vi "Create Routine.vi"(8 "error in (no error)":errorcluster, 10 "Routine":T1 {"Stop Parameters"."Response"."Byte Order" items=["Little Endian", "Big Endian"]; "Stop Parameters"."Response"."Data Type" items=["Signed", "Unsigned", "IEEE Float"]; "Stop Parameters"."Cmd"."Byte Order" items=["Little Endian", "Big Endian"]; "Stop Parameters"."Cmd"."Data Type" items=["Signed", "Unsigned", "IEEE Float"]; "Request Parameters"."Response"."Byte Order" items=["Little Endian", "Big Endian"]; "Request Parameters"."Response"."Data Type" items=["Signed", "Unsigned", "IEEE Float"]; "Request Parameters"."Cmd"."Byte Order" items=["Little Endian", "Big Endian"]; "Request Parameters"."Cmd"."Data Type" items=["Signed", "Unsigned", "IEEE Float"]; "Start Parameters"."Response"."Byte Order" items=["Little Endian", "Big Endian"]; "Start Parameters"."Response"."Data Type" items=["Signed", "Unsigned", "IEEE Float"]; "Start Parameters"."Cmd"."Byte Order" items=["Little Endian", "Big Endian"]; "Start Parameters"."Cmd"."Data Type" items=["Signed", "Unsigned", "IEEE Float"]}, 11 "Section Ptr":T4 format="%.0x") -> (0 "error out":errorcluster, 3 "Parent Ref out":T4 format="%.0x")   [LabVIEW 2015, in "Diagnostics Addon System Explorer.lvlib"]
uses:
  System Explorer/Diagnostics Addon System Explorer.lvlib
  <vilib>/NI Veristand/Custom Device API/Custom Device Item Ref.ctl
  Routine Paramaters.ctl
  Input and Output Signal Parameters.ctl
  Signal Parameters.ctl
  FG Action.ctl
  GUID Lookup.vi
  <vilib>/NI Veristand/Custom Device API/NI VeriStand - Get Item Property.vi
  <vilib>/NI Veristand/Custom Device API/Get Item Property (U32).vi
  <vilib>/NI Veristand/Custom Device API/NI VeriStand - Set Item Property.vi
  <vilib>/NI Veristand/Custom Device API/Set Item Property (U32).vi
  <vilib>/NI Veristand/Custom Device API/Custom Device API.lvlib
  Diagnostics Addon Shared.lvlib
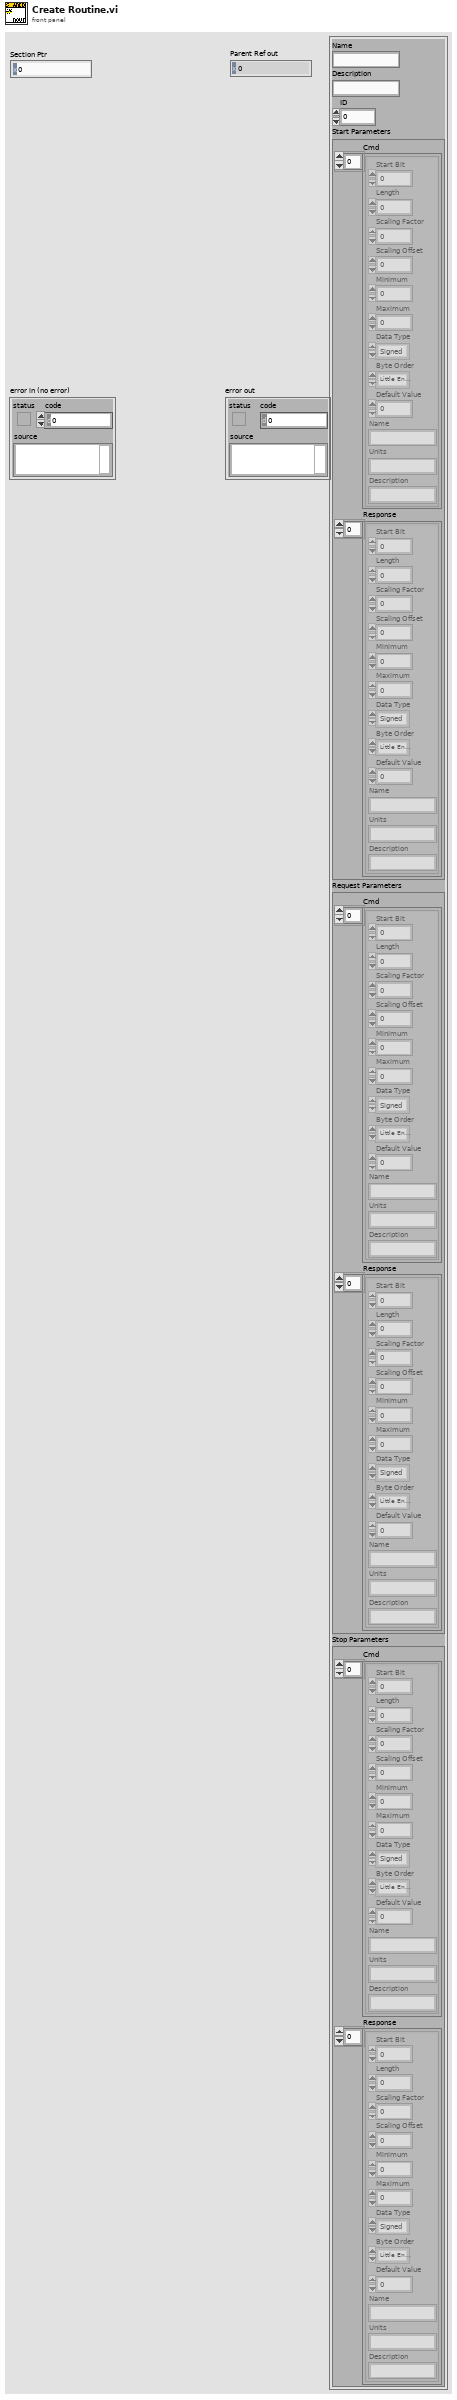
[diagram p1: front panel]
types:
  T1 = typedef "Diagnostics Addon Shared.lvlib/Routine Paramaters.ctl" = cluster{"Name":string, "Description":string, "ID":u16, "Start Parameters":T2, "Request Parameters":T2, "Stop Parameters":T2}
  T2 = typedef "Diagnostics Addon Shared.lvlib/Input and Output Signal Parameters.ctl" = cluster{"Cmd":T3[], "Response":T3[]}
  T3 = typedef "Diagnostics Addon Shared.lvlib/Signal Parameters.ctl" = cluster{"Start Bit":u8, "Length":u8, "Scaling Factor":dbl, "Scaling Offset":dbl, "Minimum":dbl, "Maximum":dbl, "Data Type":u32, "Byte Order":u32, "Default Value":dbl, "Name":string, "Units":string, "Description":string}
  T4 = typedef "Custom Device API.lvlib/Custom Device Item Ref.ctl" = u64
  T5 = typedef "Diagnostics Addon System Explorer.lvlib/FG Action.ctl" = enum16{"Get", "Set"}
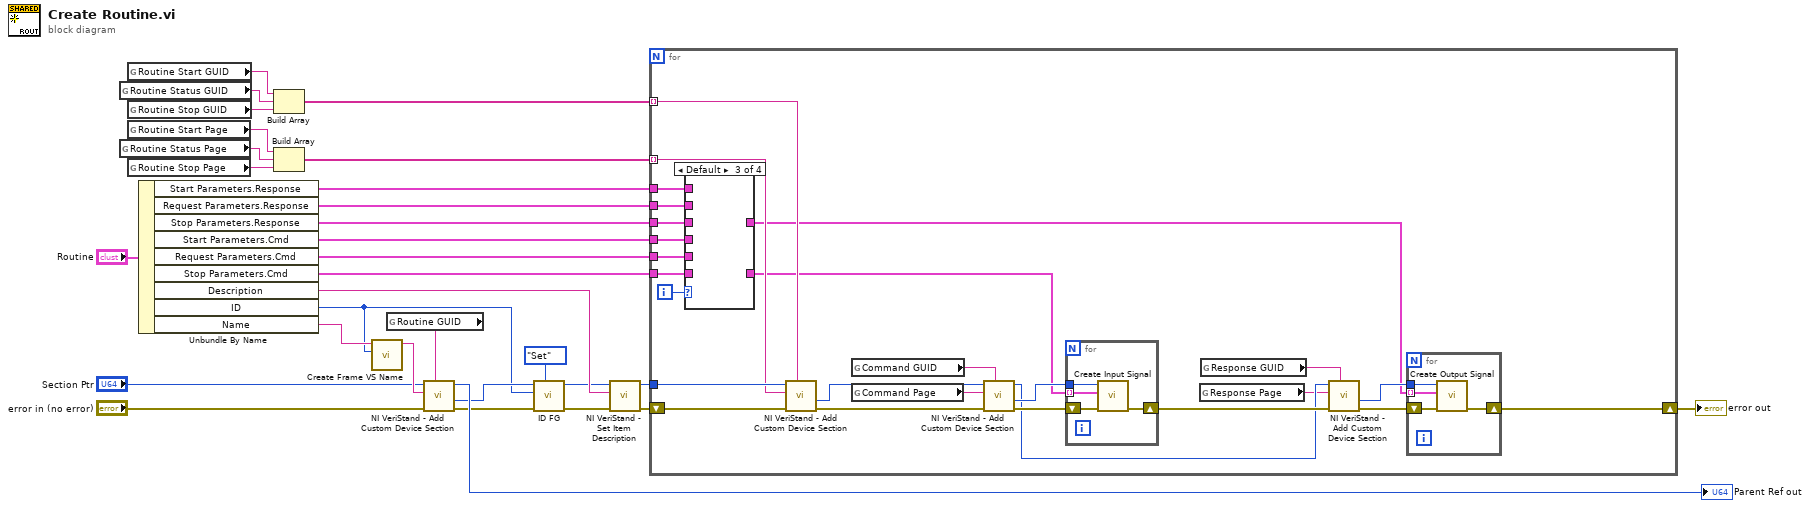
[diagram p0: block diagram]
diagram:
  n1 = global read "GUID Lookup.vi" "Routine Status GUID"() -> (w30:string)
  n2 = global read "GUID Lookup.vi" "Routine Status Page"() -> (w26:string)
  n3 = global read "GUID Lookup.vi" "Routine Start GUID"() -> (w29:string)
  n4 = global read "GUID Lookup.vi" "Routine Stop GUID"() -> (w31:string)
  n5 = global read "GUID Lookup.vi" "Routine Start Page"() -> (w27:string)
  n6 = global read "GUID Lookup.vi" "Routine Stop Page"() -> (w25:string)
  n7 = Unbundle By Name("Routine") -> ("Start Parameters.Response"=w12:T3[], "Request Parameters.Response"=w10:T3[], "Stop Parameters.Response"=w8:T3[], "Start Parameters.Cmd"=w11:T3[], "Request Parameters.Cmd"=w9:T3[], "Stop Parameters.Cmd"=w7:T3[], "Description"=w20:string, "ID"=w1:u16, "Name"=w21:string)
  n8 = Build Array(w29, w30, w31) -> (w28:string[])
  n9 = Build Array(w27, w26, w25) -> (w24:string[])
  n10 = call "Create Frame VS Name.vi"("PID Number"=w1, "PID Name"=w21) -> ("VS Name"=w23:string)  [unwired: 9 in]
  n11 = global read "GUID Lookup.vi" "Routine GUID"() -> (w17:string)
  n12 = call <vilib>:"NI VeriStand - Add Custom Device Section.vi"("GUID (Default Section)"=w17, "error in (no error)"="error in (no error)", "Section Name"=w23, "Parent Ref in"="Section Ptr") -> ("error out"=w5:errorcluster, "Section Ptr"=w4:T4, "Parent Ref out"=→"Parent Ref out":T4)  [unwired: 4 in, 1 out]
  n13 = call "ID FG.vi"("Action"=FG_Action."Set", "error in (no error)"=w5, "ID"=w1, "Device Item Ref in"=w4) -> ("error out"=w3:errorcluster, "Device Item Ref out"=w2:T4)  [unwired: 5 in, 1 out]
  n14 = call <vilib>:"NI VeriStand - Set Item Description.vi"("error in (no error)"=w3, "Description"=w20, "Item Ref in"=w2) -> ("error out"=w19:errorcluster, "Item Ref out"=w18:T4)  [unwired: 6 in, 1 out]
  n15 = for {
    tunnel: w18 -> [w56]
    shift-right: [w43] -> w14
    shift-left: w19 -> [w57]
    tunnel: w28 -> [w55] mode=indexing
    tunnel: w24 -> [w54] mode=indexing
    tunnel: w12 -> [w38]
    tunnel: w11 -> [w36]
    tunnel: w10 -> [w35]
    tunnel: w9 -> [w34]
    tunnel: w8 -> [w33]
    tunnel: w7 -> [w32]
    i -> [w40]
    n16 = case shown="Default" w40 {
      tunnel: [w59 w61 _ w63] -> w39
      tunnel: w38 -> [_ _ _ w63]
      tunnel: [w58 w60 _ w62] -> w37
      tunnel: w36 -> [_ _ _ w62]
      tunnel: w35 -> [w59 _ _ _]
      tunnel: w34 -> [w58 _ _ _]
      tunnel: w33 -> [_ w61 _ _]
      tunnel: w32 -> [_ w60 _ _]
      frame 1 {
      }
      frame 2 {
      }
      frame Default {
      }
      frame 0 {
      }
    }
    n17 = call <vilib>:"NI VeriStand - Add Custom Device Section.vi"("GUID (Default Section)"=w55, "error in (no error)"=w57, "Section Name"=w54, "Parent Ref in"=w56) -> ("error out"=w42:errorcluster, "Section Ptr"=w41:T4)  [unwired: 4 in, 2 out]
    n18 = global read "GUID Lookup.vi" "Command GUID"() -> (w45:string)
    n19 = global read "GUID Lookup.vi" "Command Page"() -> (w44:string)
    n20 = call <vilib>:"NI VeriStand - Add Custom Device Section.vi"("GUID (Default Section)"=w45, "error in (no error)"=w42, "Section Name"=w44, "Parent Ref in"=w41) -> ("error out"=w50:errorcluster, "Section Ptr"=w51:T4, "Parent Ref out"=w48:T4)  [unwired: 4 in, 1 out]
    n21 = for {
      shift-right: [w66] -> w49
      shift-left: w50 -> [w67]
      tunnel: w37 -> [w64] mode=indexing
      tunnel: w51 -> [w65]
      n22 = call "Create Input Signal.vi"("error in (no error)"=w67, "Signal Parameters"=w64, "Section Ptr"=w65) -> ("error out"=w66:errorcluster)  [unwired: 7 in, 1 out]
    }
    n23 = global read "GUID Lookup.vi" "Response Page"() -> (w47:string)
    n24 = global read "GUID Lookup.vi" "Response GUID"() -> (w46:string)
    n25 = call <vilib>:"NI VeriStand - Add Custom Device Section.vi"("GUID (Default Section)"=w46, "error in (no error)"=w49, "Section Name"=w47, "Parent Ref in"=w48) -> ("error out"=w52:errorcluster, "Section Ptr"=w53:T4)  [unwired: 4 in, 2 out]
    n26 = for {
      shift-right: [w68] -> w43
      shift-left: w52 -> [w70]
      tunnel: w39 -> [w69] mode=indexing
      tunnel: w53 -> [w71]
      n27 = call "Create Output Signal.vi"("error in (no error)"=w70, "Signal Parameters"=w69, "Section Ptr"=w71) -> ("error out"=w68:errorcluster)  [unwired: 7 in, 1 out]
    }
  }
  "error out" <- w14
